vi "Lidar Motor Controler for Controls.vi"   [LabVIEW 2009]
uses:
  Test/Lidar Chirp Global.vi
  Motor Control Global.vi
  Motor Output Global.vi
  <vilib>/Platform/TimedLoop/XDataNode/XDataNode.xnode
  <vilib>/Platform/TimedLoop/XDataNode/loadlvalarms.vi
  <vilib>/Platform/TimedLoop/XDataNode/timing_clust.ctl
  <vilib>/Platform/TimedLoop/XDataNode/nitl_modes.ctl
  <vilib>/Platform/TimedLoop/XDataNode/wakeup.ctl
  <vilib>/rvi/FXPMathLib/FxpSinAndCos/XNode/nifxpmath_SinAndCos.xnode
  <vilib>/rvi/FXPMathLib/FxpSinAndCos/subVIs/nifxpmath_SinAndCos_SimConfig.ctl
  <vilib>/rvi/FXPMathLib/FxpSinAndCos/simVIs/DllFxpSinAndCosTemp_sub.vi
  <vilib>/rvi/FXPMathLib/FxpMul/XNode/nifxpmath_Multiplier.xnode
  <vilib>/rvi/FXPMathLib/FxpMul/subVIs/nifxpmath_Mul_SimConfig.ctl
  <vilib>/fxp/LVFixedPointQuantizationPolicyTypeDef.ctl
  <vilib>/fxp/LVFixedPointOverflowPolicyTypeDef.ctl
  <vilib>/rvi/FXPMathLib/FxpMul/simVIs/DllFxpMulTemp_sub.vi
  <vilib>/rvi/FXPMathLib/FxpAdd/XNode/nifxpmath_Add.xnode
  <vilib>/rvi/FXPMathLib/FxpAdd/subVIs/nifxpmath_Add_SimConfig.ctl
  <vilib>/rvi/FXPMathLib/FxpAdd/simVIs/DllFxpAddTemp_sub.vi
  <vilib>/Platform/TimedLoop/XDataNode/XDNodeRunTimeDep.lvlib
types:
  T1 = typedef "Strict Lidar Motor Control Cluster.ctl" = cluster{"Reset Encoder":bool, "Motor Enable":bool, "Choice of Control Type":enum32{"Direct Voltage Control", "Proportional Control", "PI Control", "Custom Compensator", "PID Control", "II-PID-DD Control"}, "Choice of Oscillation":enum32{"Oscillate Voltage", "Oscillate Setpoint", "No Oscillation"}, "Choice of Compensation":enum32{"None", "Computed Torque", "Mechanical Advantage", "CT & MA "}, "Choice of Error":enum32{"Gray Error", "Lidar Error", "Kent Error", "UberKent Error"}, "Units of pi rad 18b (s-fxp-1)":cluster{"Phi_B Set Point (pi rad)":fxp<+/-,18,1>, "Phi_A Set Point (pi rad)":fxp<+/-,18,1>, "Phi_Lidar Set Point (pi rad)":fxp<+/-,18,1>, "Phi_Lidar - Phi_A":fxp<+/-,18,1>, "Phi_mass-Phi_Lidar":fxp<+/-,18,1>, "Convert (enc) to (pi rad)":fxp<+/-,18,1>, "Oscillation Frequency (pi rad per 100KHz)":fxp<+/-,18,1>}, "Units of 18b (s-fxp-1) gain":cluster{"Proportional Gain":fxp<+/-,18,1>, " Integral Gain":fxp<+/-,18,1>, "Oscillation Setpoint Amplitude":fxp<+/-,18,1>, "Gravity Compensation Gain":fxp<+/-,18,1>, "Phi_B Set Point (enc) pre-gain":fxp<+/-,18,1>, "Phi_B Set Point (pi rad) pre-gain":fxp<+/-,18,1>, "Phi_A Set Point (pi rad) pre-gain":fxp<+/-,18,1>, "Phi_Lidar Set Point (pi rad) pre-gain":fxp<+/-,18,1>, "Derivative Gain":fxp<+/-,18,1>, "Double Integral Gain":fxp<+/-,18,1>, "Second Derivative Gain":fxp<+/-,18,1>}, "Units of 20b s-fxp-5 Voltage":cluster{"Oscillation Voltage Amplitude":fxp<+/-,20,5>, "Motor Voltage":fxp<+/-,20,5>}, "Units of encoder 32b uint":cluster{"Phi_B Set Point (enc)":i32, "Lidar Encoder Cap":i32}, "Debug Args":bool[]}
  T2 = enum32{"None", "Computed Torque", "Mechanical Advantage", "CT & MA "}
  T3 = enum32{"Oscillate Voltage", "Oscillate Setpoint", "No Oscillation"}
  T4 = enum32{"Direct Voltage Control", "Proportional Control", "PI Control", "Custom Compensator", "PID Control", "II-PID-DD Control"}
  T5 = enum32{"Gray Error", "Lidar Error", "Kent Error", "UberKent Error"}
  T6 = typedef "XDNodeRunTimeDep.lvlib/timing_clust.ctl" = cluster{"Expected End [f-1]":u64, "Actual End [f-1]":u64, "Finished Late? [f-1]":bool, "Expected End [i-1]":u64, "Actual End [i-1]":u64, "Finished Late? [i-1]":bool, "Expected Start [i]":u64, "Actual Start [i]":u64, "Expected Start [f]":u64, "Actual Start [f]":u64, "Source Name":string, "Structure Name":string, "Period":i64, "Deadline":i64, "Offset":i64, "Start":i64, "Priority":i32, "Timeout":i32, "Mode":T7, "Wakeup Reason":T8, "Error":errorcluster, "Source Type":string, "Secondary Source Type":string, "Global End Time":u64, "Global Start Time":u64, "Frame Duration":u64, "Iteration Duration":u64, "Assigned CPU":i32, "I/O Scan Engine Mode":u32}
  T7 = typedef "XDNodeRunTimeDep.lvlib/nitl_modes.ctl" = enum32{"No Change", "Process missed periods, maintain original phase", "Discard missed periods, maintain original phase", "Process missed periods, ignore original phase", "Discard missed periods, ignore original phase"}
  T8 = typedef "XDNodeRunTimeDep.lvlib/wakeup.ctl" = enum32{"Normal", "Aborted", "Asynchronous wakeup", "Timing source error", "Timed loop error", "Timeout"}
  T9 = typedef "Strict Lidar Motor Indicator Cluster.ctl" = cluster{"Phi_A":fxp<+/-,18,1>, "Phi_B":fxp<+/-,18,1>, "Output Voltage":fxp<+/-,20,5>, "Phi_Lidar":fxp<+/-,18,1>, "Phi_Mass":fxp<+/-,18,1>, "MA":fxp<+/-,18,1>, "Base Output":fxp<+/-,18,1>, "Error":fxp<+/-,18,1>}
  T10 = typedef "Strict Custom Compensator.ctl" = cluster{"Zero coefficients":fxp<+/-,18,1>[], "Pole coefficients":fxp<+/-,18,1>[], "Gain":fxp<+/-,18,1>}
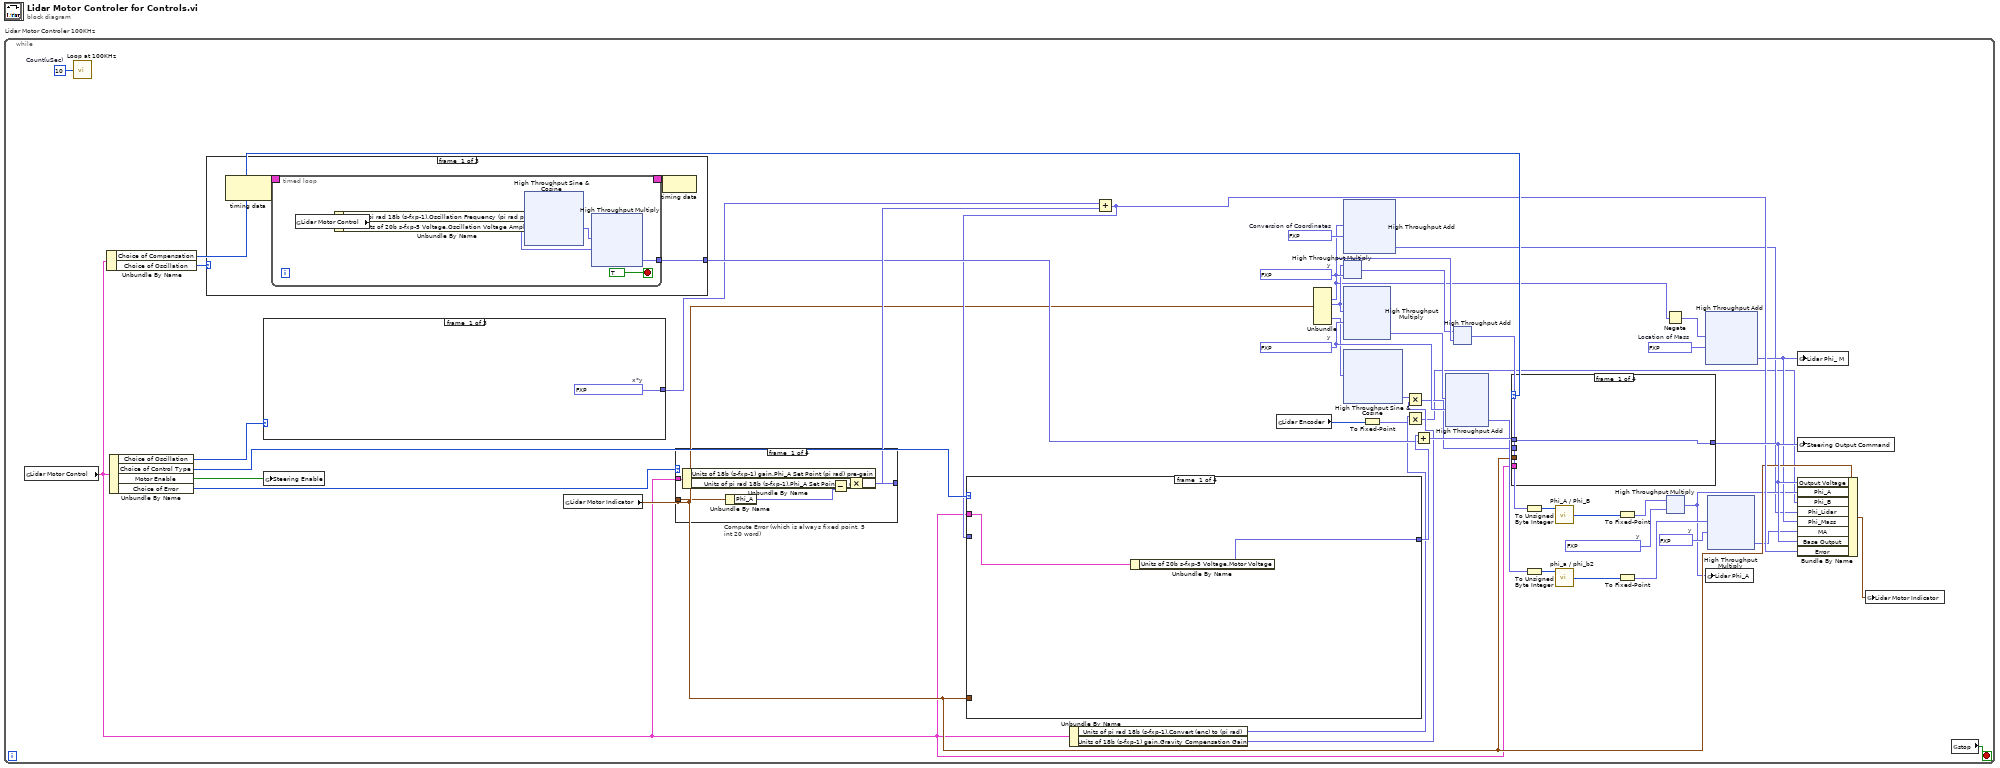
[diagram p0: block diagram]
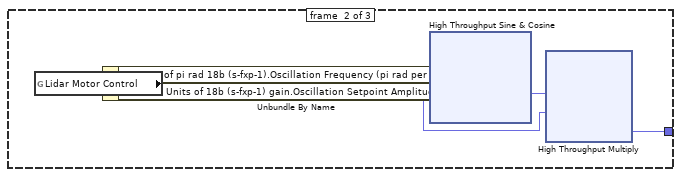
[diagram p2: hidden frame]
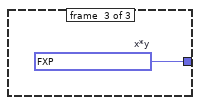
[diagram p3: hidden frame]
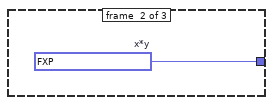
[diagram p4: hidden frame]
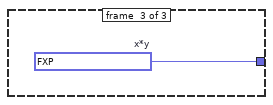
[diagram p5: hidden frame]
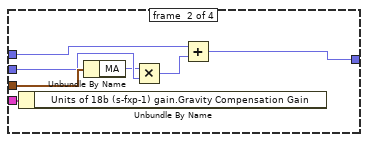
[diagram p6: hidden frame]
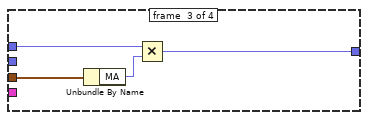
[diagram p7: hidden frame]
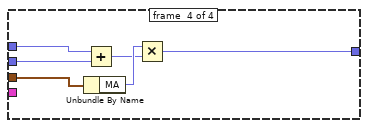
[diagram p8: hidden frame]
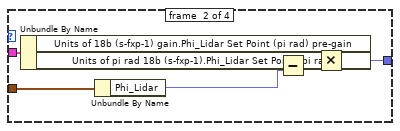
[diagram p9: hidden frame]
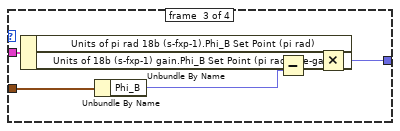
[diagram p10: hidden frame]
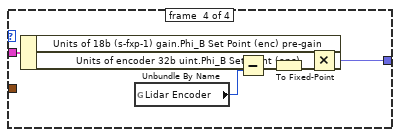
[diagram p11: hidden frame]
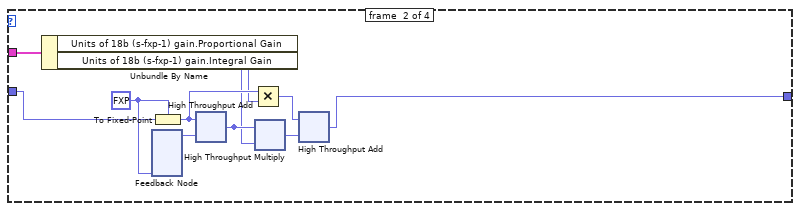
[diagram p12: hidden frame]
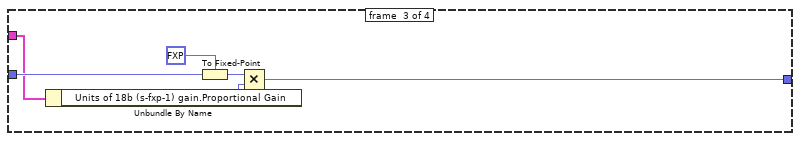
[diagram p13: hidden frame]
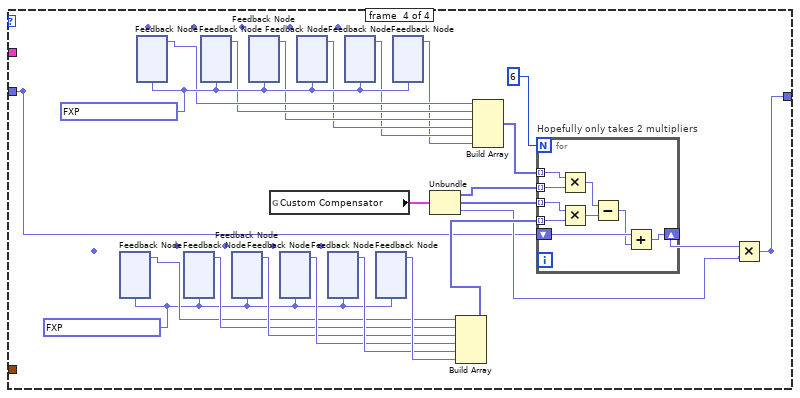
[diagram p14: hidden frame]
diagram:
  n1 = while "Lidar Motor Controler 100KHz" {
    stop <- w49 stop-if-true
    w17 = fxp<+/-,10,1> 0.3046875  # Location of Mass
    w19 = fxp<+/-,10,1> 0.103515625  # Conversion of Coordinates
    w24 = fxp<+,8,8> 128.0  # y
    w22 = fxp<+,1,-6> 0.0078125  # y
    w31 = fxp<+,8,8> 128.0  # y
    w29 = fxp<+/-,16,-3> 0.0026035308837890625  # y
    w34 = u32 10  # Count(uSec)
    n2 = global read "Motor Control Global.vi" "Lidar Motor Control"() -> (w4:T1)
    n3 = call "Loop at 100KHz"("Count(uSec)"=w34) -> ()  [unwired: 1 out]
    n4 = Unbundle By Name(w4) -> ("Choice of Compensation"=w41:T2, "Choice of Oscillation"=w40:T3)
    n5 = Unbundle By Name(w4) -> ("Choice of Oscillation"=w35:T3, "Choice of Control Type"=w48:T4, "Motor Enable"=w47:bool, "Choice of Error"=w45:T5)
    n6 = case shown="\"Oscillate Setpoint\"" w40 {
      tunnel: [w367 w436 w437] -> w38
      frame #0 {
        n7 = node-c288() -> (w366:T6)  [unwired: 1 in]
        n8 = timed-loop {
          timing: w366 -> [_]
          timing-out: [_] -> w365
          tunnel: [w369] -> w367
          stop <- TRUE stop-if-true
          n9 = global read "Motor Control Global.vi" "Lidar Motor Control"() -> (w372:T1)
          n10 = Unbundle By Name(w372) -> ("Units of pi rad 18b (s-fxp-1).Oscillation Frequency (pi rad per 100KHz)"=w371:fxp<+/-,18,1>, "Units of 20b s-fxp-5 Voltage.Oscillation Voltage Amplitude"=w370:fxp<+/-,20,5>)
          n11 = xnode ("High Throughput Sine & Cosine")("x (pi)"=w371) -> ("sin(x)"=w373:fxp<+/-,16,2>)  [unwired: 1 out]
          n12 = xnode "High Throughput Multiply"("x"=w373, "y"=w370) -> ("x*y"=w369:fxp<+/-,20,5>)
        }
        n13 = node-c288(w365) -> ()
      }
      frame #1 {
        w436 = fxp<+/-,20,5> 0.0  # x*y
      }
      frame #2 {
        w437 = fxp<+/-,20,5> 0.0  # x*y
      }
    }
    n14 = case shown="\"Oscillate Setpoint\"" w35 {
      tunnel: [w300 w301 w364] -> w36
      frame #0 {
        w300 = fxp<+/-,20,5> 0.0  # x*y
      }
      frame #1 {
        n15 = global read "Motor Control Global.vi" "Lidar Motor Control"() -> (w304:T1)
        n16 = Unbundle By Name(w304) -> ("Units of pi rad 18b (s-fxp-1).Oscillation Frequency (pi rad per 100KHz)"=w303:fxp<+/-,18,1>, "Units of 18b (s-fxp-1) gain.Oscillation Setpoint Amplitude"=w302:fxp<+/-,18,1>)
        n17 = xnode ("High Throughput Sine & Cosine")("x (pi)"=w303) -> ("sin(x)"=w305:fxp<+/-,16,2>)  [unwired: 1 out]
        n18 = xnode "High Throughput Multiply"("x"=w305, "y"=w302) -> ("x*y"=w301:fxp<+/-,20,5>)
      }
      frame #2 {
        w364 = fxp<+/-,20,5> 0.0  # x*y
      }
    }
    n19 = global write "Motor Output Global.vi" "Steering Enable"(w47) -> ()
    n20 = global read "Motor Control Global.vi" "Lidar Motor Indicator"() -> (w16:T9)
    n21 = case "Compute Error (which is always fixed point, 5 int 20 word)" shown="\"Gray Error\", Default" w45 {
      tunnel: w4 -> [w458 w469 w471 w480]
      tunnel: w16 -> [w457 w468 w472 _]
      tunnel: [w456 w463 w470 w478] -> w44
      frame #0 {
        n22 = Unbundle By Name(w458) -> ("Units of 18b (s-fxp-1) gain.Phi_A Set Point (pi rad) pre-gain"=w459:fxp<+/-,18,1>, "Units of pi rad 18b (s-fxp-1).Phi_A Set Point (pi rad)"=w462:fxp<+/-,18,1>)
        n23 = Unbundle By Name(w457) -> ("Phi_A"=w461:fxp<+/-,18,1>)
        n24 = Subtract(x=w462, y=w461) -> (x-y=w460:fxp<+/-,20,5>)
        n25 = Multiply(x=w459, y=w460) -> (x*y=w456:fxp<+/-,20,5>)
      }
      frame #1 {
        n26 = Unbundle By Name(w469) -> ("Units of 18b (s-fxp-1) gain.Phi_Lidar Set Point (pi rad) pre-gain"=w464:fxp<+/-,18,1>, "Units of pi rad 18b (s-fxp-1).Phi_Lidar Set Point (pi rad)"=w467:fxp<+/-,18,1>)
        n27 = Unbundle By Name(w468) -> ("Phi_Lidar"=w466:fxp<+/-,18,1>)
        n28 = Subtract(x=w467, y=w466) -> (x-y=w465:fxp<+/-,20,5>)
        n29 = Multiply(x=w464, y=w465) -> (x*y=w463:fxp<+/-,20,5>)
      }
      frame #2 {
        n30 = Unbundle By Name(w471) -> ("Units of pi rad 18b (s-fxp-1).Phi_B Set Point (pi rad)"=w473:fxp<+/-,18,1>, "Units of 18b (s-fxp-1) gain.Phi_B Set Point (pi rad) pre-gain"=w476:fxp<+/-,18,1>)
        n31 = Unbundle By Name(w472) -> ("Phi_B"=w475:fxp<+/-,18,1>)
        n32 = Subtract(x=w476, y=w475) -> (x-y=w474:fxp<+/-,20,5>)
        n33 = Multiply(x=w473, y=w474) -> (x*y=w470:fxp<+/-,20,5>)
      }
      frame #3 {
        n34 = Unbundle By Name(w480) -> ("Units of 18b (s-fxp-1) gain.Phi_B Set Point (enc) pre-gain"=w481:fxp<+/-,18,1>, "Units of encoder 32b uint.Phi_B Set Point (enc)"=w483:i32)
        n35 = global read "Motor Control Global.vi" "Lidar Encoder"() -> (w479:i32)
        n36 = Subtract(x=w483, y=w479) -> (x-y=w482:i32)
        n37 = To Fixed-Point(number=w482) -> (fixed-point=w477:fxp<+/-,32,32>)  [unwired: 1 in]
        n38 = Multiply(x=w481, y=w477) -> (x*y=w478:fxp<+/-,20,5>)
      }
    }
    n39 = Unbundle By Name(w4) -> ("Units of pi rad 18b (s-fxp-1).Convert (enc) to (pi rad)"=w2:fxp<+/-,18,1>, "Units of 18b (s-fxp-1) gain.Gravity Compensation Gain"=w7:fxp<+/-,18,1>)
    n40 = Add(x=w36, y=w44) -> (x+y=w37:fxp<+/-,20,5>)
    n41 = case shown="\"PI Control\"" w48 {
      tunnel: [w484 w489 w582 w585] -> w43
      tunnel: w37 -> [_ w490 w581 w587]
      tunnel: w4 -> [w485 w488 w580 _]
      tunnel: w16 -> [_ _ _ _]
      frame #0 {
        n42 = Unbundle By Name(w485) -> ("Units of 20b s-fxp-5 Voltage.Motor Voltage"=w484:fxp<+/-,20,5>)
      }
      frame #1 {
        w494 = fxp<+/-,20,5> 0.0 ("fixed-point type")
        n43 = Unbundle By Name(w488) -> ("Units of 18b (s-fxp-1) gain.Proportional Gain"=w487:fxp<+/-,18,1>, "Units of 18b (s-fxp-1) gain.Integral Gain"=w486:fxp<+/-,18,1>)
        n44 = feedback #1(w494) -> (w493:fxp<+/-,20,5>)
        n45 = To Fixed-Point(fixed-point type=w494, number=w490) -> (fixed-point=w492:fxp<+/-,20,5>)
        n46 = xnode "High Throughput Add"("x"=w492, "y"=w493) -> ("x+y"=w495:fxp<+/-,20,5>)
        n47 = Multiply(x=w492, y=w487) -> (x*y=w491:fxp<+/-,20,5>)
        n48 = xnode "High Throughput Multiply"("x"=w495, "y"=w486) -> ("x*y"=w496:fxp<+/-,20,5>)
        n49 = xnode "High Throughput Add"("x"=w491, "y"=w496) -> ("x+y"=w489:fxp<+/-,20,5>)
      }
      frame #2 {
        n50 = Unbundle By Name(w580) -> ("Units of 18b (s-fxp-1) gain.Proportional Gain"=w579:fxp<+/-,18,1>)
        n51 = To Fixed-Point(fixed-point type=fxp<+/-,20,5> 0.0, number=w581) -> (fixed-point=w583:fxp<+/-,20,5>)
        n52 = Multiply(x=w583, y=w579) -> (x*y=w582:fxp<+/-,20,5>)
      }
      frame #3 {
        w594 = fxp<+/-,20,5> 0.0
        w607 = fxp<+/-,20,5> 0.0
        n53 = feedback #2(w594) -> (w595:fxp<+/-,20,5>)
        n54 = feedback #3(w607) -> (w606:fxp<+/-,20,5>)
        n55 = feedback #4(w594) -> (w596:fxp<+/-,20,5>)
        n56 = feedback #5(w607) -> (w605:fxp<+/-,20,5>)
        n57 = feedback #6(w594) -> (w597:fxp<+/-,20,5>)
        n58 = feedback #7(w607) -> (w604:fxp<+/-,20,5>)
        n59 = global read "Motor Control Global.vi" "Custom Compensator"() -> (w608:T10)
        n60 = feedback #8(w594) -> (w598:fxp<+/-,20,5>)
        n61 = feedback #9(w607) -> (w603:fxp<+/-,20,5>)
        n62 = feedback #10(w594) -> (w599:fxp<+/-,20,5>)
        n63 = feedback #11(w607) -> (w602:fxp<+/-,20,5>)
        n64 = feedback #12(w594) -> (w600:fxp<+/-,20,5>)
        n65 = feedback #13(w607) -> (w601:fxp<+/-,20,5>)
        n66 = Unbundle(w608) -> ("Zero coefficients"=w590:fxp<+/-,18,1>[], "Pole coefficients"=w589:fxp<+/-,18,1>[], "Gain"=w588:fxp<+/-,18,1>)
        n67 = Build Array(w595, w596, w597, w598, w599, w600) -> (w592:fxp<+/-,20,5>[])
        n68 = Build Array(w606, w605, w604, w603, w602, w601) -> (w593:fxp<+/-,20,5>[])
        n69 = for "Hopefully only takes 2 multipliers" {
          N: 6 -> [_]
          tunnel: w593 -> [w617] mode=indexing
          tunnel: w592 -> [w613] mode=indexing
          tunnel: w590 -> [w616] mode=indexing
          tunnel: w589 -> [w614] mode=indexing
          shift-right: [w609] -> w586
          shift-left: w587 -> [w611]
          n70 = Multiply(x=w617, y=w616) -> (x*y=w615:fxp<+/-,20,5>)
          n71 = Multiply(x=w614, y=w613) -> (x*y=w612:fxp<+/-,20,5>)
          n72 = Subtract(x=w615, y=w612) -> (x-y=w610:fxp<+/-,20,5>)
          n73 = Add(x=w611, y=w610) -> (x+y=w609:fxp<+/-,20,5>)
        }
        n74 = Multiply(x=w586, y=w588) -> (x*y=w585:fxp<+/-,20,5>)
      }
    }
    n75 = global read "Motor Control Global.vi" "Lidar Encoder"() -> (w5:i32)
    n76 = Unbundle(w16) -> ("Output Voltage"=w13:fxp<+/-,20,5>, "Phi_Lidar"=w14:fxp<+/-,18,1>, "Base Output"=w11:fxp<+/-,18,1>)  [unwired: 5 out]
    n77 = xnode "High Throughput Add"("x"=w13, "y"=w19) -> ("x+y"=w9:fxp<+/-,10,1>)
    n78 = xnode "High Throughput Multiply"("x"=w14, "y"=w31) -> ("x*y"=w30:fxp<+/-,8,8>)
    n79 = xnode "High Throughput Multiply"("x"=w14, "y"=w24) -> ("x*y"=w23:fxp<+/-,8,8>)
    n80 = xnode "High Throughput Sine & Cosine"("x (pi)"=w11) -> ("cos(x)"=w8:fxp<+/-,16,2>)  [unwired: 1 out]
    n81 = To Fixed-Point(number=w5) -> (fixed-point=w1:fxp<+/-,32,32>)  [unwired: 1 in]
    n82 = Multiply(x=w8, y=w7) -> (x*y=w6:fxp<+/-,34,3>)
    n83 = Multiply(x=w2, y=w1) -> (x*y=w3:fxp<+/-,10,1>)
    n84 = Add(x=w43, y=w38) -> (x+y=w39:fxp<+/-,20,5>)
    n85 = xnode "High Throughput Add"("x"=w23, "y"=w24) -> ("x+y"=w25:fxp<+,8,8>)
    n86 = xnode "High Throughput Add"("x"=w30, "y"=w31) -> ("x+y"=w32:fxp<+,8,8>)
    n87 = case shown="\"CT & MA \"" w41 {
      tunnel: [w438 w444 w446 w450] -> w42
      tunnel: w39 -> [w438 w445 w448 w453]
      tunnel: w16 -> [_ w443 w449 w455]
      tunnel: w4 -> [_ w442 _ _]
      tunnel: w6 -> [_ w441 _ w452]
      frame #0 {
      }
      frame #1 {
        n88 = Unbundle By Name(w442) -> ()  [unwired: 1 out]
        n89 = Unbundle By Name(w443) -> ("MA"=w440:fxp<+/-,18,1>)
        n90 = Multiply(x=w440, y=w441) -> (x*y=w439:fxp<+/-,20,5>)
        n91 = Add(x=w445, y=w439) -> (x+y=w444:fxp<+/-,20,5>)
      }
      frame #2 {
        n92 = Unbundle By Name(w449) -> ("MA"=w447:fxp<+/-,18,1>)
        n93 = Multiply(x=w448, y=w447) -> (x*y=w446:fxp<+/-,20,5>)
      }
      frame #3 {
        n94 = Unbundle By Name(w455) -> ("MA"=w454:fxp<+/-,18,1>)
        n95 = Add(x=w453, y=w452) -> (x+y=w451:fxp<+/-,20,5>)
        n96 = Multiply(x=w454, y=w451) -> (x*y=w450:fxp<+/-,20,5>)
      }
    }
    n97 = To Unsigned Byte Integer(number=w32) -> (unsigned 8bit integer=w33:u8)
    n98 = To Unsigned Byte Integer(number=w25) -> (unsigned 8bit integer=w26:u8)
    n99 = call "Phi_A / Phi_B"("address"=w33) -> ("data out"=w27:i8)  [unwired: 8 in]
    n100 = call "phi_a / phi_b2"("address"=w26) -> ("data out"=w20:i8)  [unwired: 8 in]
    n101 = To Fixed-Point(number=w27) -> (fixed-point=w28:fxp<+/-,8,8>)  [unwired: 1 in]
    n102 = To Fixed-Point(number=w20) -> (fixed-point=w21:fxp<+/-,8,8>)  [unwired: 1 in]
    n103 = Negate(x=w13) -> (-x=w18:fxp<+/-,21,6>)
    n104 = xnode "High Throughput Multiply"("x"=w28, "y"=w29) -> ("x*y"=w10:fxp<+/-,10,1>)
    n105 = xnode "High Throughput Add"("x"=w18, "y"=w17) -> ("x+y"=w12:fxp<+/-,10,1>)
    n106 = global write "Lidar Chirp Global.vi" "Lidar Phi_A"(w10) -> ()
    n107 = xnode "High Throughput Multiply"("x"=w21, "y"=w22) -> ("x*y"=w15:fxp<+/-,8,1>)
    n108 = global write "Lidar Chirp Global.vi" "Lidar Phi_ M"(w12) -> ()
    n109 = global write "Motor Output Global.vi" "Steering Output Command"(w42) -> ()
    n110 = Bundle By Name(cluster=w16, "Output Voltage"=w42, "Phi_A"=w10, "Phi_B"=w3, "Phi_Lidar"=w9, "Phi_Mass"=w12, "MA"=w15, "Base Output"=w42, "Error"=w37) -> (w46:T9)
    n111 = global write "Motor Control Global.vi" "Lidar Motor Indicator"(w46) -> ()
    n112 = global read "Motor Control Global.vi" "stop"() -> (w49:bool)
  }
